vi "EnqueueSettings.vi"(8 "error in (no error)":errorcluster, 9 "Data":variant, 10 "Message":T1, 11 "SettingsQueue":refnum<queue>) -> (0 "error out":errorcluster, 3 "queue out":refnum<queue>)   [LabVIEW 2019, in "Settings.lvlib"]
uses:
  Settings.lvlib
  CTL_SettingsMessage.ctl
  CTL_MessageCluster.ctl
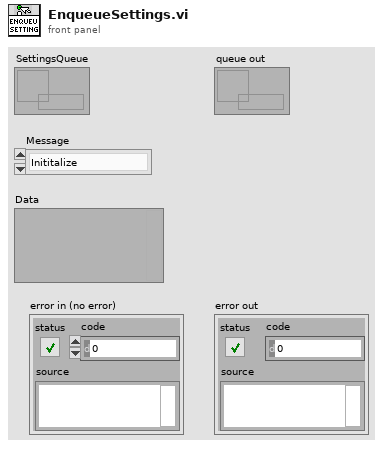
[diagram p1: front panel]
types:
  T1 = typedef "Settings.lvlib/CTL_SettingsMessage.ctl" = enum16{"Inititalize", "Idle", "LoadSettings", "SaveSettings", "Exit"}
  T2 = typedef "Settings.lvlib/CTL_MessageCluster.ctl" = cluster{"Message":T1, "Data":variant}
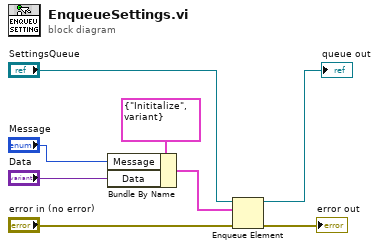
[diagram p0: block diagram]
diagram:
  n1 = Bundle By Name(cluster=T2 {"Message"=enum."Inititalize", "Data"=variant} ("element"), "Message"="Message", "Data"="Data") -> (w6:T2)
  n2 = Enqueue Element(queue="SettingsQueue", element=w6, error in (no error)="error in (no error)") -> (queue out=→"queue out":refnum<queue>, error out=→"error out":errorcluster)  [unwired: 1 in, 1 out]
